vi "REPORT.Main.vi"(4 "Delimiter":string="\t", 9 "Test IN":T22 {"Test Registros"."Read W/R" format="%04x"; "Test Registros"."Pattern W/R" format="%04x"; "Test Registros"."Read Default" format="%04x"; "Test Registros"."Pattern Default" format="%04x"}) -> (1 "Report OUT":string="[SUMMARY TEST]\r\n--------------------------------------------------------------------------------\r\n[BACK PANEL INFORMATION]\r\nReference Card\tBPV3-S4815000xxxx\r\nUnique ID\t00000014FFD5\r\nDate\t2016.04.14-10.29.08\r\n[SUMMARY TEST RESULT]\r\nTest Trigger\tFAIL\r\nTest L1 Fan Out\tNO DATA\r\nTest Delay\tNO DATA\r\nTest Noise\tNO DATA\r\n\r\n[RESULT TEST TRIGGER]\r\n--------------------------------------------------------------------------------\r\n[CONFIG TRIGGER]\r\nLOOPS TRIGGER\t2\r\nWAIT PPS TRIGGER\t12\r\n[PATTERN TRIGGER]\r\nPPS\tCLKEXT\tTRG L1\tSPARES1\tBUSY\tTRGTYPE0\tTRGTYPE0\tTRGTYPE0\tTRGCONFIG\r\n0C\t0098967F\tC350\tC350\tC350\tC350\tC350\tC350\tC350\r\n[FINAL RESULT TEST TRIGGER]\r\n\tRUN0\tRUN1\tRUN2\tRUN3\tRUN4\tRUN5\tRUN6\r\nLOOP 0\tOK\tERROR\tOK\tOK\tOK\tOK\tOK\r\nLOOP 1\tOK\tOK\tOK\tOK\tOK\tOK\tOK\r\n[VALUES TRIGGER]\r\nRUN\tLOOP\tGEO\tPPS\tCLKEXT\tTRG L1\tSPARES1\tBUSY\tTRGTYPE0\tTRGTYPE1\tTRGTYPE2\tTRGCONFIG\tRESULT\r\n0\t0\t0\t0C\t0098967F\tC350\tC350\tC350\tC350\tC350\tC350\tC350\tOK\r\n0\t0\t1\t0C\t0098967F\tC350\tC350\tC350\tC350\tC350\tC350\tC350\tOK\r\n0\t0\t2\t0C\t0098967F\tC350\tC350\tC350\tC350\tC350\tC350\tC350\tOK\r\n0\t0\t3\t0C\t0098967F\tC350\tC350\tC350\tC350\tC350\tC350\tC350\tOK\r\n0\t0\t4\t0C\t0098967F\tC350\tC350\tC350\tC350\tC350\tC350\tC350\tOK\r\n0\t0\t5\t0C\t0098967F\tC350\tC350\tC350\tC350\tC350\tC350\tC350\tOK\r\n0\t0\t6\t0C\t0098967F\tC350\tC350\tC350\tC350\tC350\tC350\tC350\tOK\r\n0\t1\t0\t0C\t0098967F\tC350\tC350\tC350\tC350\tC350\tC350\tC350\tOK\r\n0\t1\t1\t0C\t0098967F\tC350\tC350\tC350\tC350\tC350\tC350\tC350\tOK\r\n0\t1\t2\t0C\t0098967F\tC350\tC350\tC350\tC350\tC350\tC350\tC350\tOK\r\n0\t1\t3\t0C\t0098967F\tC350\tC350\tC350\tC350\tC350\tC350\tC350\tOK\r\n0\t1\t4\t0C\t0098967F\tC350\tC350\tC350\tC350\tC350\tC350\tC350\tOK\r\n0\t1\t5\t0C\t0098967F\tC350\tC350\tC350\tC350\tC350\tC350\tC350\tOK\r\n0\t1\t6\t0C\t0098967F\tC350\tC350\tC350\tC350\tC350\tC350\tC350\tOK\r\n1\t0\t0\t0C\t0098967F\tC350\tC350\tC350\tC350\tC350\tC350\tC350\tOK\r\n1\t0\t1\t0C\t0098967F\tC350\tC350\tC350\tC350\tC350\tC350\tC350\tOK\r\n1\t0\t2\t0C\t0098967F\tC350\tC350\tC350\tC350\tC350\tC350\tC350\tOK\r\n1\t0\t3\t0C\t0098967F\tC350\tC350\tC350\tC350\tC350\tC350\t0000\tOK\r\n1\t0\t4\t0C\t0098967F\t9322\t9322\t9322\t9322\t9322\t9322\t0000\tERROR\r\n1\t0\t5\t0C\t0098967F\tC350\tC350\tC350\tC350\tC350\tC350\t0000\tOK\r\n1\t0\t6\t0C\t0098967F\tC350\tC350\tC350\tC350\tC350\tC350\tC350\tOK\r\n1\t1\t0\t0C\t0098967F\tC350\tC350\tC350\tC350\tC350\tC350\tC350\tOK\r\n1\t1\t1\t0C\t0098967F\tC350\tC350\tC350\tC350\tC350\tC350\tC350\tOK\r\n1\t1\t2\t0C\t0098967F\tC350\tC350\tC350\tC350\tC350\tC350\tC350\tOK\r\n1\t1\t3\t0C\t0098967F\tC350\tC350\tC350\tC350\tC350\tC350\t0000\tOK\r\n1\t1\t4\t0C\t0098967F\tC350\tC350\tC350\tC350\tC350\tC350\t0000\tOK\r\n1\t1\t5\t0C\t0098967F\tC350\tC350\tC350\tC350\tC350\tC350\t0000\tOK\r\n1\t1\t6\t0C\t0098967F\tC350\tC350\tC350\tC350\tC350\tC350\tC350\tOK\r\n2\t0\t0\t0C\t0098967F\tC350\tC350\tC350\tC350\tC350\tC350\tC350\tOK\r\n2\t0\t1\t0C\t0098967F\tC350\tC350\tC350\tC350\tC350\tC350\tC350\tOK\r\n2\t0\t2\t0C\t0098967F\tC350\tC350\tC350\tC350\tC350\tC350\tC350\tOK\r\n2\t0\t3\t0C\t0098967F\tC350\tC350\tC350\tC350\tC350\tC350\tC350\tOK\r\n2\t0\t4\t0C\t0098967F\tC350\tC350\tC350\tC350\tC350\tC350\t0000\tOK\r\n2\t0\t5\t0C\t0098967F\tC350\tC350\tC350\tC350\tC350\tC350\t0000\tOK\r\n2\t0\t6\t0C\t0098967F\tC350\tC350\tC350\tC350\tC350\tC350\t0000\tOK\r\n2\t1\t0\t0C\t0098967F\tC350\tC350\tC350\tC350\tC350\tC350\tC350\tOK\r\n2\t1\t1\t0C\t0098967F\tC350\tC350\tC350\tC350\tC350\tC350\tC350\tOK\r\n2\t1\t2\t0C\t0098967F\tC350\tC350\tC350\tC350\tC350\tC350\tC350\tOK\r\n2\t1\t3\t0C\t0098967F\tC350\tC350\tC350\tC350\tC350\tC350\tC350\tOK\r\n2\t1\t4\t0C\t0098967F\tC350\tC350\tC350\tC350\tC350\tC350\t0000\tOK\r\n2\t1\t5\t0C\t0098967F\tC350\tC350\tC350\tC350\tC350\tC350\t0000\tOK\r\n2\t1\t6\t0C\t0098967F\tC350\tC350\tC350\tC350\tC350\tC350\t0000\tOK\r\n3\t0\t0\t0C\t0098967F\tC350\tC350\tC350\tC350\tC350\tC350\tC350\tOK\r\n3\t0\t1\t0C\t0098967F\tC350\tC350\tC350\tC350\tC350\tC350\t0000\tOK\r\n3\t0\t2\t0C\t0098967F\tC350\tC350\tC350\tC350\tC350\tC350\tC350\tOK\r\n3\t0\t3\t0C\t0098967F\tC350\tC350\tC350\tC350\tC350\tC350\tC350\tOK\r\n3\t0\t4\t0C\t0098967F\tC350\tC350\tC350\tC350\tC350\tC350\tC350\tOK\r\n3\t0\t5\t0C\t0098967F\tC350\tC350\tC350\tC350\tC350\tC350\t0000\tOK\r\n3\t0\t6\t0C\t0098967F\tC350\tC350\tC350\tC350\tC350\tC350\t0000\tOK\r\n3\t1\t0\t0C\t0098967F\tC350\tC350\tC350\tC350\tC350\tC350\tC350\tOK\r\n3\t1\t1\t0C\t0098967F\tC350\tC350\tC350\tC350\tC350\tC350\t0000\tOK\r\n3\t1\t2\t0C\t0098967F\tC350\tC350\tC350\tC350\tC350\tC350\tC350\tOK\r\n3\t1\t3\t0C\t0098967F\tC350\tC350\tC350\tC350\tC350\tC350\tC350\tOK\r\n3\t1\t4\t0C\t0098967F\tC350\tC350\tC350\tC350\tC350\tC350\tC350\tOK\r\n3\t1\t5\t0C\t0098967F\tC350\tC350\tC350\tC350\tC350\tC350\t0000\tOK\r\n3\t1\t6\t0C\t0098967F\tC350\tC350\tC350\tC350\tC350\tC350\t0000\tOK\r\n4\t0\t0\t0C\t0098967F\tC350\tC350\tC350\tC350\tC350\tC350\tC350\tOK\r\n4\t0\t1\t0C\t0098967F\tC350\tC350\tC350\tC350\tC350\tC350\t0000\tOK\r\n4\t0\t2\t0C\t0098967F\tC350\tC350\tC350\tC350\tC350\tC350\t0000\tOK\r\n4\t0\t3\t0C\t0098967F\tC350\tC350\tC350\tC350\tC350\tC350\tC350\tOK\r\n4\t0\t4\t0C\t0098967F\tC350\tC350\tC350\tC350\tC350\tC350\tC350\tOK\r\n4\t0\t5\t0C\t0098967F\tC350\tC350\tC350\tC350\tC350\tC350\tC350\tOK\r\n4\t0\t6\t0C\t0098967F\tC350\tC350\tC350\tC350\tC350\tC350\t0000\tOK\r\n4\t1\t0\t0C\t0098967F\tC350\tC350\tC350\tC350\tC350\tC350\tC350\tOK\r\n4\t1\t1\t0C\t0098967F\tC350\tC350\tC350\tC350\tC350\tC350\t0000\tOK\r\n4\t1\t2\t0C\t0098967F\tC350\tC350\tC350\tC350\tC350\tC350\t0000\tOK\r\n4\t1\t3\t0C\t0098967F\tC350\tC350\tC350\tC350\tC350\tC350\tC350\tOK\r\n4\t1\t4\t0C\t0098967F\tC350\tC350\tC350\tC350\tC350\tC350\tC350\tOK\r\n4\t1\t5\t0C\t0098967F\tC350\tC350\tC350\tC350\tC350\tC350\tC350\tOK\r\n4\t1\t6\t0C\t0098967F\tC350\tC350\tC350\tC350\tC350\tC350\t0000\tOK\r\n5\t0\t0\t0C\t0098967F\tC350\tC350\tC350\tC350\tC350\tC350\tC350\tOK\r\n5\t0\t1\t0C\t0098967F\tC350\tC350\tC350\tC350\tC350\tC350\t0000\tOK\r\n5\t0\t2\t0C\t0098967F\tC350\tC350\tC350\tC350\tC350\tC350\t0000\tOK\r\n5\t0\t3\t0C\t0098967F\tC350\tC350\tC350\tC350\tC350\tC350\t0000\tOK\r\n5\t0\t4\t0C\t0098967F\tC350\tC350\tC350\tC350\tC350\tC350\tC350\tOK\r\n5\t0\t5\t0C\t0098967F\tC350\tC350\tC350\tC350\tC350\tC350\tC350\tOK\r\n5\t0\t6\t0C\t0098967F\tC350\tC350\tC350\tC350\tC350\tC350\tC350\tOK\r\n5\t1\t0\t0C\t0098967F\tC350\tC350\tC350\tC350\tC350\tC350\tC350\tOK\r\n5\t1\t1\t0C\t0098967F\tC350\tC350\tC350\tC350\tC350\tC350\t0000\tOK\r\n5\t1\t2\t0C\t0098967F\tC350\tC350\tC350\tC350\tC350\tC350\t0000\tOK\r\n5\t1\t3\t0C\t0098967F\tC350\tC350\tC350\tC350\tC350\tC350\t0000\tOK\r\n5\t1\t4\t0C\t0098967F\tC350\tC350\tC350\tC350\tC350\tC350\tC350\tOK\r\n5\t1\t5\t0C\t0098967F\tC350\tC350\tC350\tC350\tC350\tC350\tC350\tOK\r\n5\t1\t6\t0C\t0098967F\tC350\tC350\tC350\tC350\tC350\tC350\tC350\tOK\r\n6\t0\t0\t0C\t0098967F\tC350\tC350\tC350\tC350\tC350\tC350\tC350\tOK\r\n6\t0\t1\t0C\t0098967F\tC350\tC350\tC350\tC350\tC350\tC350\tC350\tOK\r\n6\t0\t2\t0C\t0098967F\tC350\tC350\tC350\tC350\tC350\tC350\t0000\tOK\r\n6\t0\t3\t0C\t0098967F\tC350\tC350\tC350\tC350\tC350\tC350\t0000\tOK\r\n6\t0\t4\t0C\t0098967F\tC350\tC350\tC350\tC350\tC350\tC350\t0000\tOK\r\n6\t0\t5\t0C\t0098967F\tC350\tC350\tC350\tC350\tC350\tC350\tC350\tOK\r\n6\t0\t6\t0C\t0098967F\tC350\tC350\tC350\tC350\tC350\tC350\tC350\tOK\r\n6\t1\t0\t0C\t0098967F\tC350\tC350\tC350\tC350\tC350\tC350\tC350\tOK\r\n6\t1\t1\t0C\t0098967F\tC350\tC350\tC350\tC350\tC350\tC350\tC350\tOK\r\n6\t1\t2\t0C\t0098967F\tC350\tC350\tC350\tC350\tC350\tC350\t0000\tOK\r\n6\t1\t3\t0C\t0098967F\tC350\tC350\tC350\tC350\tC350\tC350\t0000\tOK\r\n6\t1\t4\t0C\t0098967F\tC350\tC350\tC350\tC350\tC350\tC350\t0000\tOK\r\n6\t1\t5\t0C\t0098967F\tC350\tC350\tC350\tC350\tC350\tC350\tC350\tOK\r\n6\t1\t6\t0C\t0098967F\tC350\tC350\tC350\tC350\tC350\tC350\tC350\tOK\r\n\r\n", 3 "Test OUT":T1={"Info"={"Ref. Card"="", "Unique ID"="", "Date"=timestamp(0 s since 1904-01-01), "User"="", "Path Salida"=path "", "Level"=0}, "Print"={"Volcar Registro"=FALSE, "Tipo de Informe"=enum."Corto"}, "VISA"={"VISA Power Supply"="", "Visa Signal Gen"="", "IDN Power Supply"="", "IDN Signal Gene"=""}, "Cluster Card"=[], "Test Trigger"={"Test Trigger?"=FALSE, "Loop Trigger"=0, "Status Cards"=[], "Result.Graphics"=[], "Result.Binary"=[], "T. Trigger OK?"=FALSE, "Wait Counters"=0, "Pattern Trigger"={"PPS"=0, "CLKEXT"=0, "TRG L1"=0, "SPARES1"=0, "BUSY"=0, "TRGTYPE0"=0, "TRGTYPE1"=0, "TRGTYPE2"=0, "TRGCONFIG"=0}, "Counters.Values"=[], "Counters.Binary"=[], "Status CTA"={"Date/Hour"=timestamp(0 s since 1904-01-01), "Temp CTA0..CTA 6"=[]}, "Num Run"=0, "Run Start"=0, "Run Stop"=0}, "Test Fanout"={"Test Fanout?"=FALSE, "Loop Fanout"=0, "Status Card"=[], "Result.Graphis"=[], "Result.Binary"=[], "T. Fanout OK?"=FALSE, "V test"=enum."100 mV", "Max Diff"=0.0, "Pattern Asics"=[], "Asic.Bin"=[], "Asic.Value"=[], "Asic.diff"=[], "Status CTA"={"Date/Hour"=timestamp(0 s since 1904-01-01), "Temp CTA0..CTA 6"=[]}}, "Test Delays"={"Test Delays?"=FALSE, "Loop Delay"=0, "Status Card"=[], "Result.Graphis"=[], "Result.Binary"=[], "T. Delay OK?"=FALSE, "Step Fine"=0, "Delay.value"=[], "Step Coarse"=0, "Pattern Delay"={"Slope CMax"=0.0, "Intercep CMax"=0.0, "Slope Cmin"=0.0, "Intercep Cmin"=0.0, "Slope FMax"=0.0, "Intercep FMax"=0.0, "Slope Fmin"=0.0, "Intercep Fmin"=0.0}, "Status CTA"={"Date/Hour"=timestamp(0 s since 1904-01-01), "Temp CTA0..CTA 6"=[]}, "Run Start"=0, "Run Stop"=0, "Delay.value Plane"=[], "Delay.value Offset"=[]}, "Test Noise"={"Test Noise?"=FALSE, "Loop Noise"=0, "Status Card"=[], "Result.Graphis"=[], "Result.Binary"=[], "T. Noise OK?"=FALSE, "Inicio TH"=0.0, "Final TH"=0.0, "Max Noise"=0.0, "Asic.Noise"=[], "Asic.Vthmin"=[], "Asic.Vtmax"=[], "Valores Geo - Loop"=[], "Status CTA"={"Date/Hour"=timestamp(0 s since 1904-01-01), "Temp CTA0..CTA 6"=[]}}, "Info machine"={"SO"="", "SO Name"="", "SO Ver"="", "SO Build"="", "CPU"="", "APP"="", "APP YEAR"="", "APP ver"="", "APP User"="", "APP Serail"="", "MAC"=[], "PC NAME"=[], "PC IP"=[], "BIOS MANU"="", "BIOS NAME"="", "BIOS SERIAL"="", "BOARD MANU"="", "BOARD NAME"="", "BOARD SERIAL"="", "Driver Version"="", "Library Version"=""}, "BP info START"={"Date/Hour"=timestamp(0 s since 1904-01-01), "Temp Geo0..Geo 6"=[], "V Back Plane"=0.0, "I Back Plane"=0.0, "V Cta Test"=0.0, "I Cta Test"=0.0}, "CTA info Start"={"Date/Hour"=timestamp(0 s since 1904-01-01), "Temp CTA0..CTA 6"=[]}, "BP info STOP"={"Date/Hour"=timestamp(0 s since 1904-01-01), "Temp Geo0..Geo 6"=[], "V Back Plane"=0.0, "I Back Plane"=0.0, "V Cta Test"=0.0, "I Cta Test"=0.0}, "CTA info STOP"={"Date/Hour"=timestamp(0 s since 1904-01-01), "Temp CTA0..CTA 6"=[]}} {"Test Noise"."Asic.Vtmax" format="%#_6p"; "Test Noise"."Asic.Vthmin" format="%#_6p"; "Test Noise"."Max Noise" format="%#_6p"; "Test Noise"."Final TH" format="%#_6p"; "Test Noise"."Inicio TH" format="%#_6p"; "Test Noise"."Asic.Noise" format="%#_6p"; "Test Noise"."Result.Graphis" items=["No Test", "Test Ok", "Test Error", "En proceso", "Error programa"]; "Test Delays"."Result.Graphis" items=["No Test", "Test Ok", "Test Error", "En proceso", "Error programa"]; "Cluster Card"."ID CTA" format="%012x"; "Cluster Card"."Tº CTA" format="%.2f"; "Cluster Card"."Ver CTA" format="%02x"; "Cluster Card"."Ver BP" format="%04x"; "Cluster Card"."IDTEST" format="%012x"; "Cluster Card"."Tº BP" format="%.2f"; "Cluster Card"."ID BP" format="%012x"; "Test Fanout"."Asic.diff" format="%#_6p"; "Test Fanout"."Max Diff" format="%#_6p"; "Test Fanout"."Pattern Asics" format="%#_6p"; "Test Fanout"."Asic.Value" format="%#_6p"; "Test Fanout"."Asic.Bin" format="%02x"; "Test Fanout"."Result.Graphis" items=["No Test", "Test Ok", "Test Error", "En proceso", "Error programa"]; "Test Trigger"."Pattern Trigger"."TRGCONFIG" format="%04x"; "Test Trigger"."Pattern Trigger"."TRGTYPE2" format="%04x"; "Test Trigger"."Pattern Trigger"."TRGTYPE1" format="%04x"; "Test Trigger"."Pattern Trigger"."TRGTYPE0" format="%04x"; "Test Trigger"."Pattern Trigger"."BUSY" format="%04x"; "Test Trigger"."Pattern Trigger"."SPARES1" format="%04x"; "Test Trigger"."Pattern Trigger"."PPS" format="%02x"; "Test Trigger"."Pattern Trigger"."CLKEXT" format="%06x"; "Test Trigger"."Pattern Trigger"."TRG L1" format="%04x"; "Test Trigger"."Result.Graphics" items=["No Test", "Test Ok", "Test Error", "En proceso", "Error programa"]; "Test Trigger"."Counters.Binary" format="%02x"})   [LabVIEW 2009]
uses:
  _CONTROL.Check test small.ctl
  _CONTROL.Check test 2d small.ctl
  _CONTROL.Patron validacion relojes.ctl
  _CONTROL.Reultado Ensayo Triggers.ctl
  _CONTROL.Vout 81130A.ctl
  _CONTROL.Resultado Ensayo L1fanout.ctl
  _CONTROL.Cluster x1 status back plane.ctl
  _CONTROL.Cluster x7 status back pLane.ctl
  _CONTROL.Resultado Ensayo Delay.ctl
  _CONTROL.Resultado Ensayo Ruido.ctl
  _CONTROL.Test VISA.ctl
  _CONTROL.Test info.ctl
  _CONTROL.Test print.ctl
  _CONTROL.TEST.ctl
  _CONTROL.Status Back PLane.ctl
  _CONTROL.informacion pc.ctl
  _control.Delay.Pattern.ctl
  _CONTROL.Status CTA.ctl
  _CONTROL.Delay.value.ctl
  _CONTROL.Delay.value back plane.ctl
  _CONTROL.Delay.value OFFSET.ctl
  Test_result.ctl
  test_result fvasic.ctl
panel:
  out "CSV OUT":string
  # "CLUSTER TEST"
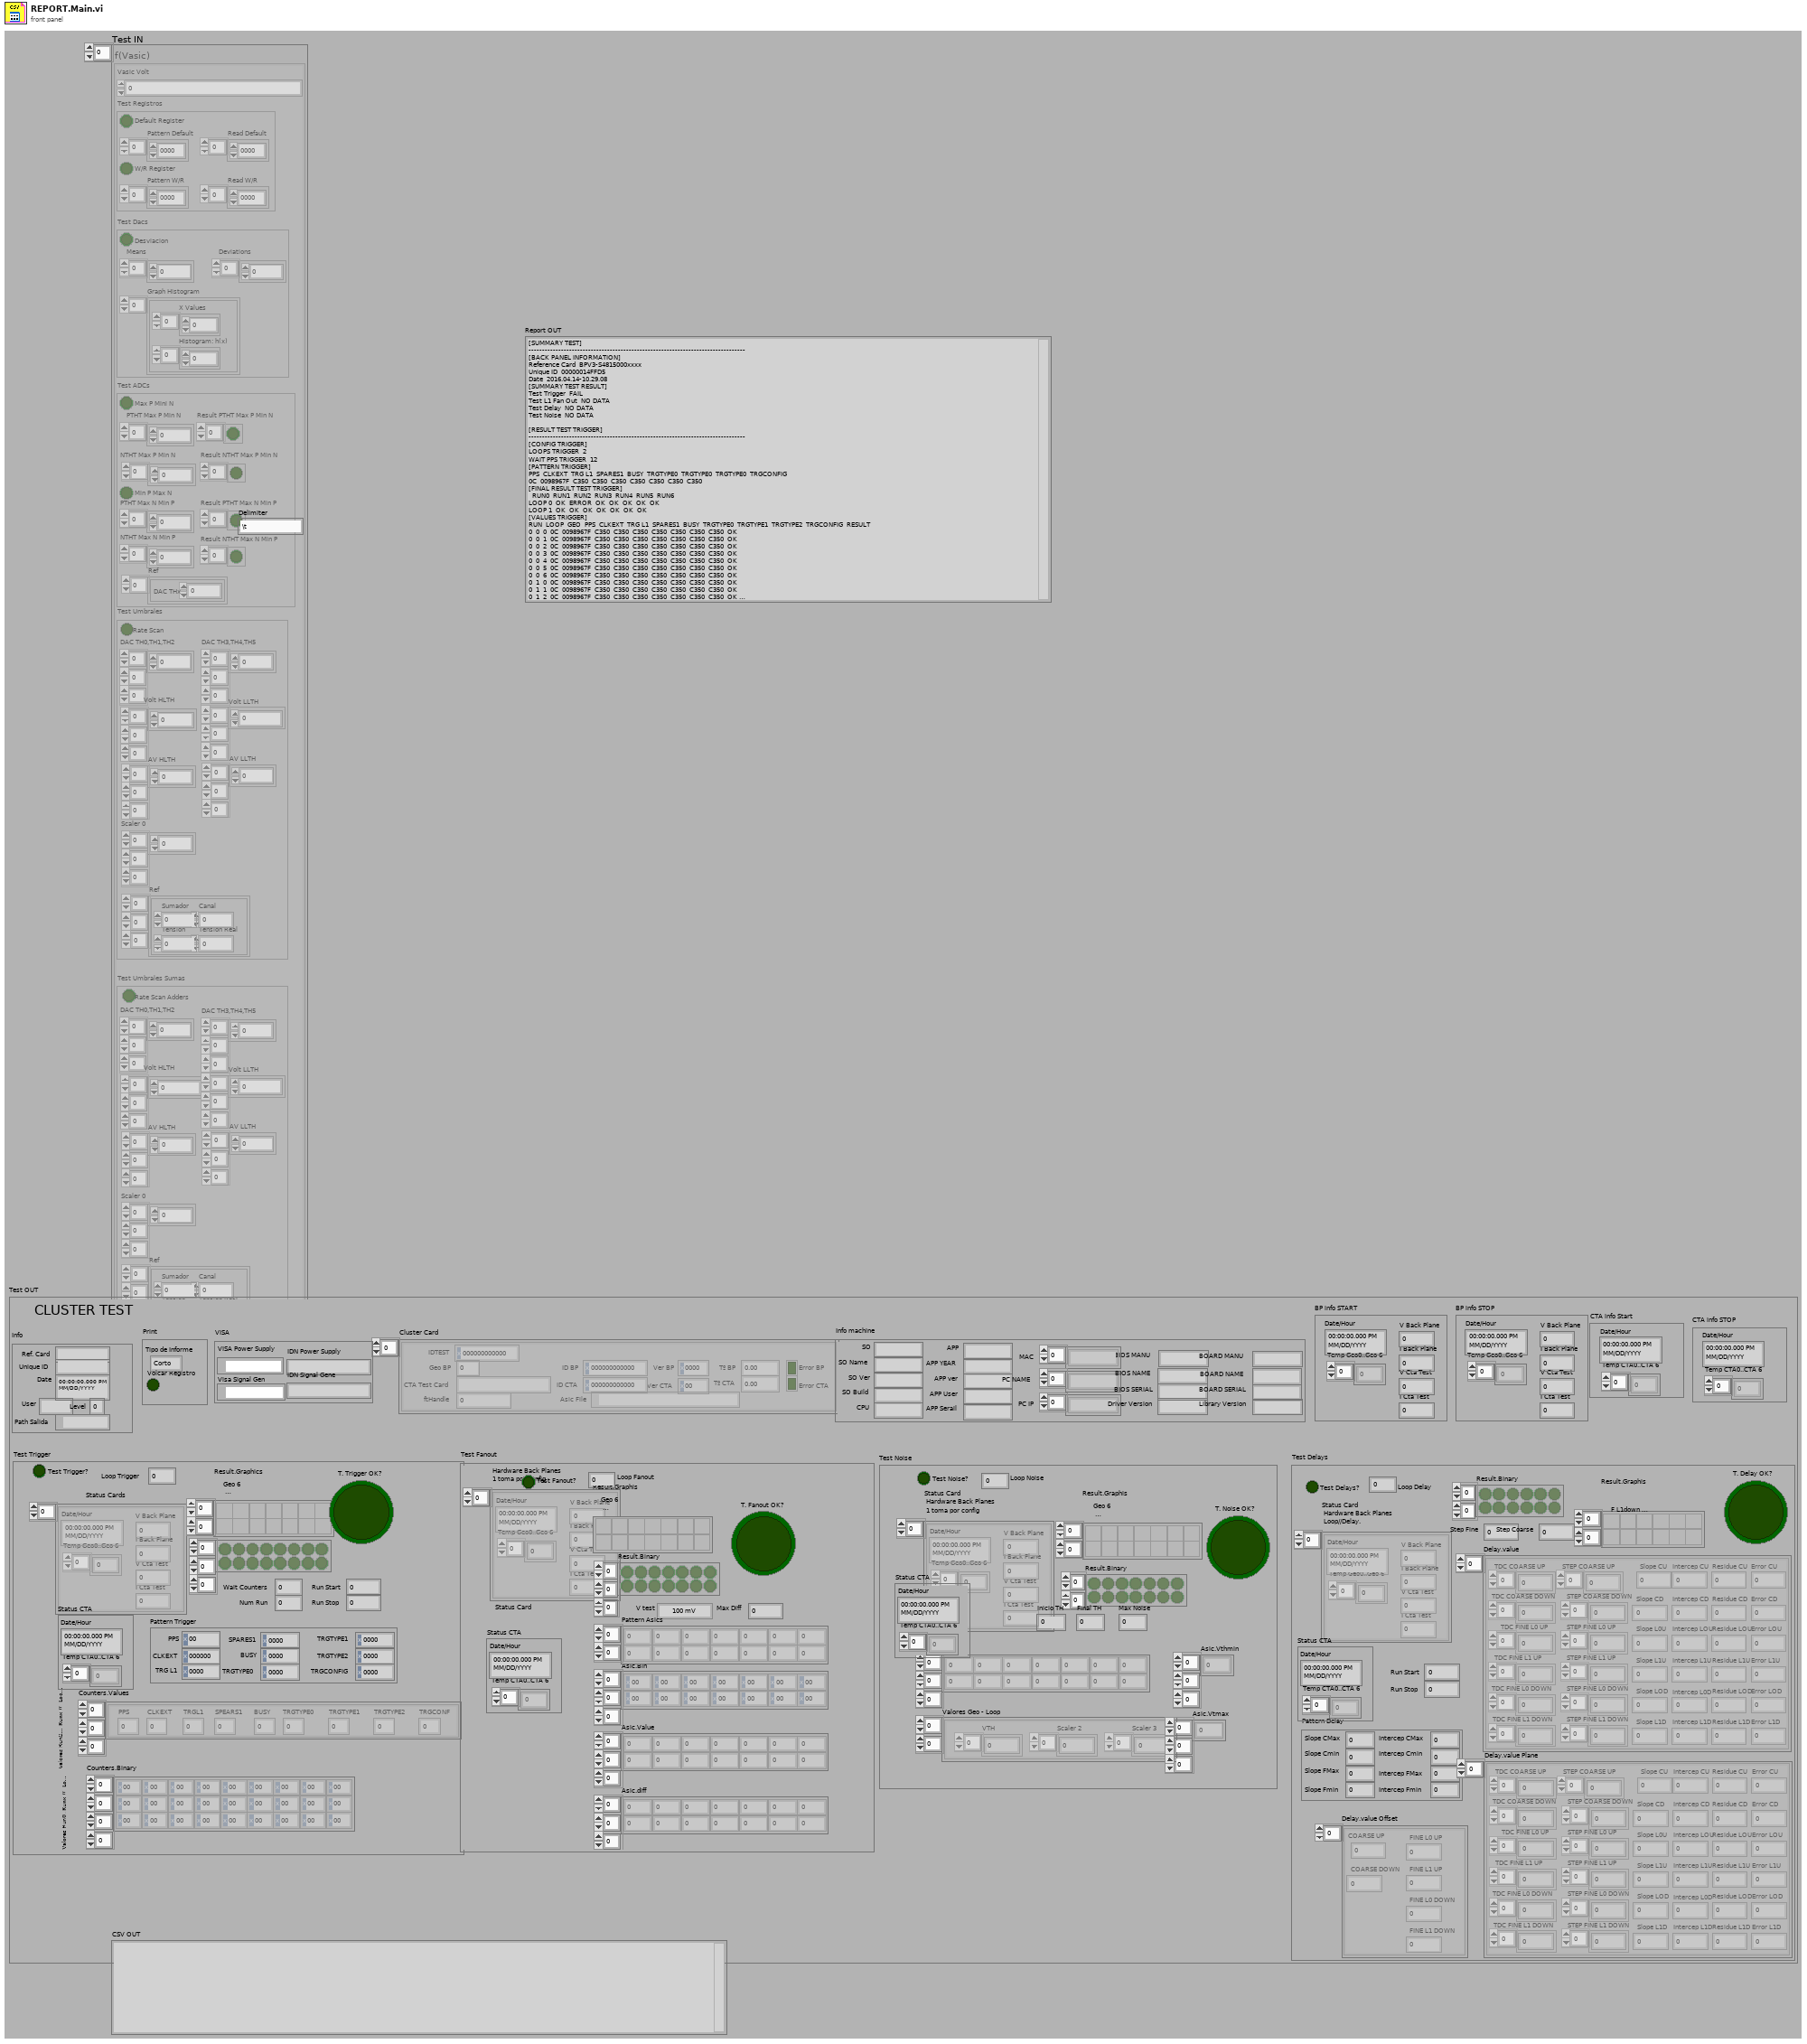
[diagram p1: front panel]
types:
  T1 = typedef "_CONTROL.TEST.ctl" = cluster{"Info":T2, "Print":T3, "VISA":T4, "Cluster Card":T5, "Test Trigger":T7, "Test Fanout":T13, "Test Delays":T15, "Test Noise":T20, "Info machine":T21, "BP info START":T8, "CTA info Start":T12, "BP info STOP":T8, "CTA info STOP":T12}
  T2 = typedef "_CONTROL.Test info.ctl" = cluster{"Ref. Card":string, "Unique ID":string, "Date":timestamp, "User":string, "Path Salida":path, "Level":i32}
  T3 = typedef "_CONTROL.Test print.ctl" = cluster{"Volcar Registro":bool, "Tipo de Informe":enum16{"Corto", "Completo"}}
  T4 = typedef "_CONTROL.Test VISA.ctl" = cluster{"VISA Power Supply":refnum<k15>, "Visa Signal Gen":refnum<visa-resource-name>, "IDN Power Supply":string, "IDN Signal Gene":string}
  T5 = typedef "_CONTROL.Cluster x7 status back pLane.ctl" = T6[]
  T6 = typedef "_CONTROL.Cluster x1 status back plane.ctl" = cluster{"Geo BP":u16, "CTA Test Card":string, "ftHandle":u32, "Error CTA":bool, "Error BP":bool, "ID BP":u64, "Tº BP":sgl, "Asic File":path, "IDTEST":u64, "Ver BP":u16, "Ver CTA":u8, "Tº CTA":sgl, "ID CTA":u64}
  T7 = typedef "_CONTROL.Reultado Ensayo Triggers.ctl" = cluster{"Test Trigger?":bool, "Loop Trigger":u8, "Status Cards":T8[], "Result.Graphics":T9, "Result.Binary":bool[][][], "T. Trigger OK?":bool, "Wait Counters":u8, "Pattern Trigger":T11, "Counters.Values":cluster{"PPS":u8, "CLKEXT":u32, "TRGL1":u16, "SPEARS1":u16, "BUSY":u16, "TRGTYPE0":u16, "TRGTYPE1":u16, "TRGTYPE2":u16, "TRGCONF":u16}[][][], "Counters.Binary":u8[][][][], "Status CTA":T12, "Num Run":u8, "Run Start":i32, "Run Stop":i32}
  T8 = typedef "_CONTROL.Status Back PLane.ctl" = cluster{"Date/Hour":timestamp, "Temp Geo0..Geo 6":sgl[], "V Back Plane":dbl, "I Back Plane":dbl, "V Cta Test":dbl, "I Cta Test":dbl}
  T9 = typedef "_CONTROL.Check test 2d small.ctl" = T10[][]
  T10 = typedef "_CONTROL.Check test small.ctl" = u16
  T11 = typedef "_CONTROL.Patron validacion relojes.ctl" = cluster{"PPS":u8, "CLKEXT":u32, "TRG L1":u16, "SPARES1":u16, "BUSY":u16, "TRGTYPE0":u16, "TRGTYPE1":u16, "TRGTYPE2":u16, "TRGCONFIG":u16}
  T12 = typedef "_CONTROL.Status CTA.ctl" = cluster{"Date/Hour":timestamp, "Temp CTA0..CTA 6":sgl[]}
  T13 = typedef "_CONTROL.Resultado Ensayo L1fanout.ctl" = cluster{"Test Fanout?":bool, "Loop Fanout":u8, "Status Card":T8[], "Result.Graphis":T9, "Result.Binary":bool[][][], "T. Fanout OK?":bool, "V test":T14, "Max Diff":dbl, "Pattern Asics":dbl[][], "Asic.Bin":u8[][][], "Asic.Value":dbl[][][], "Asic.diff":dbl[][][], "Status CTA":T12}
  T14 = typedef "_CONTROL.Vout 81130A.ctl" = enum16{"Off 0 mV", "100 mV", "200 mV", "300 mV", "400 mV", "500 mV", "600 mV", "700 mV", "800 mV", "900 mV", "1000 mV"}
  T15 = typedef "_CONTROL.Resultado Ensayo Delay.ctl" = cluster{"Test Delays?":bool, "Loop Delay":u8, "Status Card":T8[], "Result.Graphis":T9, "Result.Binary":bool[][], "T. Delay OK?":bool, "Step Fine":u8, "Delay.value":T16[], "Step Coarse":u8, "Pattern Delay":T17, "Status CTA":T12, "Run Start":i32, "Run Stop":i32, "Delay.value Plane":T18[], "Delay.value Offset":T19[]}
  T16 = typedef "_CONTROL.Delay.value.ctl" = cluster{"TDC COARSE UP":dbl[], "STEP COARSE UP":u16[], "Slope CU":dbl, "Intercep CU":dbl, "Residue CU":dbl, "Error CU":dbl, "TDC COARSE DOWN":dbl[], "STEP COARSE DOWN":u16[], "Slope CD":dbl, "Intercep CD":dbl, "Residue CD":dbl, "Error CD":dbl, "TDC FINE L0 UP":dbl[], "STEP FINE L0 UP":u16[], "Slope L0U":dbl, "Intercep LOU":dbl, "Residue LOU":dbl, "Error LOU":dbl, "TDC FINE L1 UP":dbl[], "STEP FINE L1 UP":u16[], "Slope L1U":dbl, "Intercep L1U":dbl, "Residue L1U":dbl, "Error L1U":dbl, "TDC FINE L0 DOWN":dbl[], "STEP FINE L0 DOWN":u16[], "Slope LOD":dbl, "Intercep L0D":dbl, "Residue LOD":dbl, "Error LOD":dbl, "TDC FINE L1 DOWN":dbl[], "STEP FINE L1 DOWN":u16[], "Slope L1D":dbl, "Intercep L1D":dbl, "Residue L1D":dbl, "Error L1D":dbl}
  T17 = typedef "_control.Delay.Pattern.ctl" = cluster{"Slope CMax":dbl, "Intercep CMax":dbl, "Slope Cmin":dbl, "Intercep Cmin":dbl, "Slope FMax":dbl, "Intercep FMax":dbl, "Slope Fmin":dbl, "Intercep Fmin":dbl}
  T18 = typedef "_CONTROL.Delay.value back plane.ctl" = cluster{"TDC COARSE UP":dbl[], "STEP COARSE UP":u16[], "Slope CU":dbl, "Intercep CU":dbl, "Residue CU":dbl, "Error CU":dbl, "TDC COARSE DOWN":dbl[], "STEP COARSE DOWN":u16[], "Slope CD":dbl, "Intercep CD":dbl, "Residue CD":dbl, "Error CD":dbl, "TDC FINE L0 UP":dbl[], "STEP FINE L0 UP":u16[], "Slope L0U":dbl, "Intercep LOU":dbl, "Residue LOU":dbl, "Error LOU":dbl, "TDC FINE L1 UP":dbl[], "STEP FINE L1 UP":u16[], "Slope L1U":dbl, "Intercep L1U":dbl, "Residue L1U":dbl, "Error L1U":dbl, "TDC FINE L0 DOWN":dbl[], "STEP FINE L0 DOWN":u16[], "Slope LOD":dbl, "Intercep L0D":dbl, "Residue LOD":dbl, "Error LOD":dbl, "TDC FINE L1 DOWN":dbl[], "STEP FINE L1 DOWN":u16[], "Slope L1D":dbl, "Intercep L1D":dbl, "Residue L1D":dbl, "Error L1D":dbl}
  T19 = typedef "_CONTROL.Delay.value OFFSET.ctl" = cluster{"COARSE UP":dbl, "COARSE DOWN":dbl, "FINE L0 UP":dbl, "FINE L1 UP":dbl, "FINE L0 DOWN":dbl, "FINE L1 DOWN":dbl}
  T20 = typedef "_CONTROL.Resultado Ensayo Ruido.ctl" = cluster{"Test Noise?":bool, "Loop Noise":u8, "Status Card":T8[], "Result.Graphis":T9, "Result.Binary":bool[][], "T. Noise OK?":bool, "Inicio TH":dbl, "Final TH":dbl, "Max Noise":dbl, "Asic.Noise":dbl[][][], "Asic.Vthmin":dbl[][][], "Asic.Vtmax":dbl[][][], "Valores Geo - Loop":cluster{"VTH":dbl[], "Scaler 2":u16[], "Scaler 3":u16[]}[][], "Status CTA":T12}
  T21 = typedef "_CONTROL.informacion pc.ctl" = cluster{"SO":string, "SO Name":string, "SO Ver":string, "SO Build":string, "CPU":string, "APP":string, "APP YEAR":string, "APP ver":string, "APP User":string, "APP Serail":string, "MAC":string[], "PC NAME":string[], "PC IP":string[], "BIOS MANU":string, "BIOS NAME":string, "BIOS SERIAL":string, "BOARD MANU":string, "BOARD NAME":string, "BOARD SERIAL":string, "Driver Version":string, "Library Version":string}
  T22 = typedef "Test_result.ctl" = T23[]
  T23 = typedef "test_result fvasic.ctl" = cluster{"Vasic Volt":i32, "Test Registros":cluster{"Default Register":bool, "Pattern Default":u16[], "Read Default":u16[], "W/R Register":bool, "Pattern W/R":u16[], "Read W/R":u16[]}, "Test Dacs":cluster{"Desviacion":bool, "Means":dbl[], "Deviations":dbl[], "Graph Histogram":cluster{"X Values":dbl[], "Histogram: h(x)":i32[]}[]}, "Test ADCs":cluster{"Max P Mini N":bool, "PTHT Max P Min N":dbl[], "Result PTHT Max P Min N":bool[], "NTHT Max P Min N":dbl[], "Result NTHT Max P Min N":bool[], "Min P Max N":bool, "PTHT Max N Min P":dbl[], "Result PTHT Max N Min P":bool[], "NTHT Max N Min P":dbl[], "Result NTHT Max N Min P":bool[], "Ref":cluster{"DAC THx":u8}[]}, "Test Umbrales":cluster{"Rate Scan":bool, "DAC TH0,TH1,TH2":u16[][][], "Volt HLTH":dbl[][][], "AV HLTH":dbl[][][], "DAC TH3,TH4,TH5":u16[][][], "Volt LLTH":dbl[][][], "AV LLTH":dbl[][][], "Scaler 0":u16[][][], "Ref":cluster{"Sumador":u8, "Canal":u8, "Tension":u8, "Tension Real":dbl}[][][]}, "Test Umbrales Sumas":cluster{"Rate Scan Adders":bool, "DAC TH0,TH1,TH2":u16[][][], "Volt HLTH":dbl[][][], "AV HLTH":dbl[][][], "DAC TH3,TH4,TH5":u16[][][], "Volt LLTH":dbl[][][], "AV LLTH":dbl[][][], "Scaler 0":u16[][][], "Ref":cluster{"Sumador":u8, "Canal":u8, "Tension":u8, "Tension Real":dbl}[][][]}, "Test Offset Analog":cluster{"Offset Analog":bool, "V ADDOUT":dbl[][], "Ref":cluster{"Sumador":u8, "Canal":u8}[][]}, "Test Offset Digital":cluster{"Offset Digital":bool, "Scaler 1":u16[][][], "LVDS 0 HL":bool[][][], "DAC TH0,TH1,TH2":u16[][][], "Volt HLTH":dbl[][][], "Scaler 2":u16[][][], "LVDS 1 LL":bool[][][], "DAC TH3,TH4,TH5":u16[][][], "Volt LLTH":dbl[][][], "Scaler 0":u16[][][], "Ref":cluster{"Sumador":u8, "Canal":u8}[][]}}
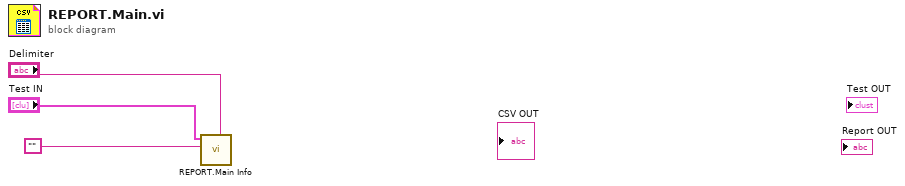
[diagram p0: block diagram]
diagram:
  n1 = call "REPORT.Main Info.vi"("Delimiter"="Delimiter", "CSV In"="", "Test IN"="Test IN") -> ()  [unwired: 8 in, 1 out]
